vi "test_mean_map_filtered_M_stripped.vi"() -> ()   [LabVIEW 2009]
doc: "Copyright (C) 2009, Stepan A. Baranov\nweb: http://www.OCTLab.org/\nemail: stepan@baranov.su"
uses:
  OCTLib.dll
panel:
  out "min":dbl format="%0.2f"
  out "max":dbl format="%0.2f"
  out "version":string
  out "name":string
  out "error out":errorcluster
  out "offset":i32
  out "strip size":i32
  out "A-scan size":i32
  out "# of A-scans":i32
  in  "Small/Big":bool
  out "loop #":i32
  out "RSM_STAT time":u32
  out "LabView time":u32
  out "RSM_STAT Array":dbl[][](array[numeric])
  out "LabView Array":dbl[][](array[numeric])
  in  "stop":bool
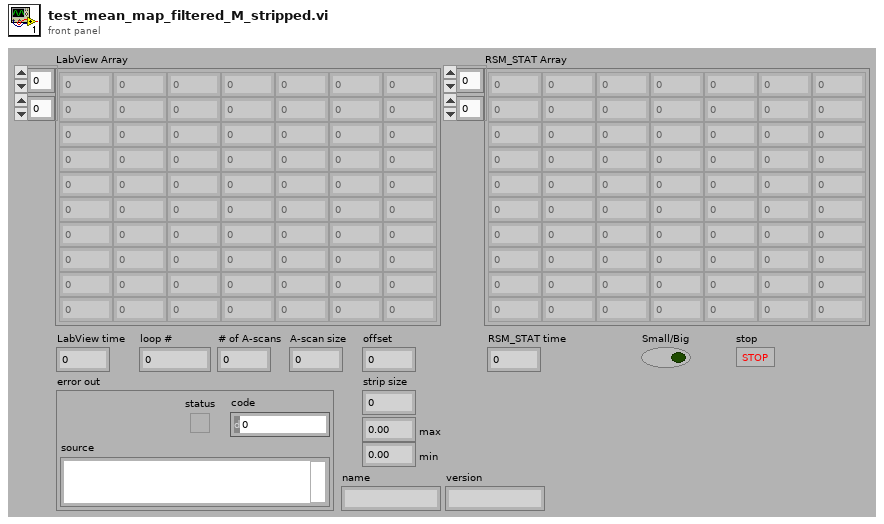
[diagram p1: front panel]
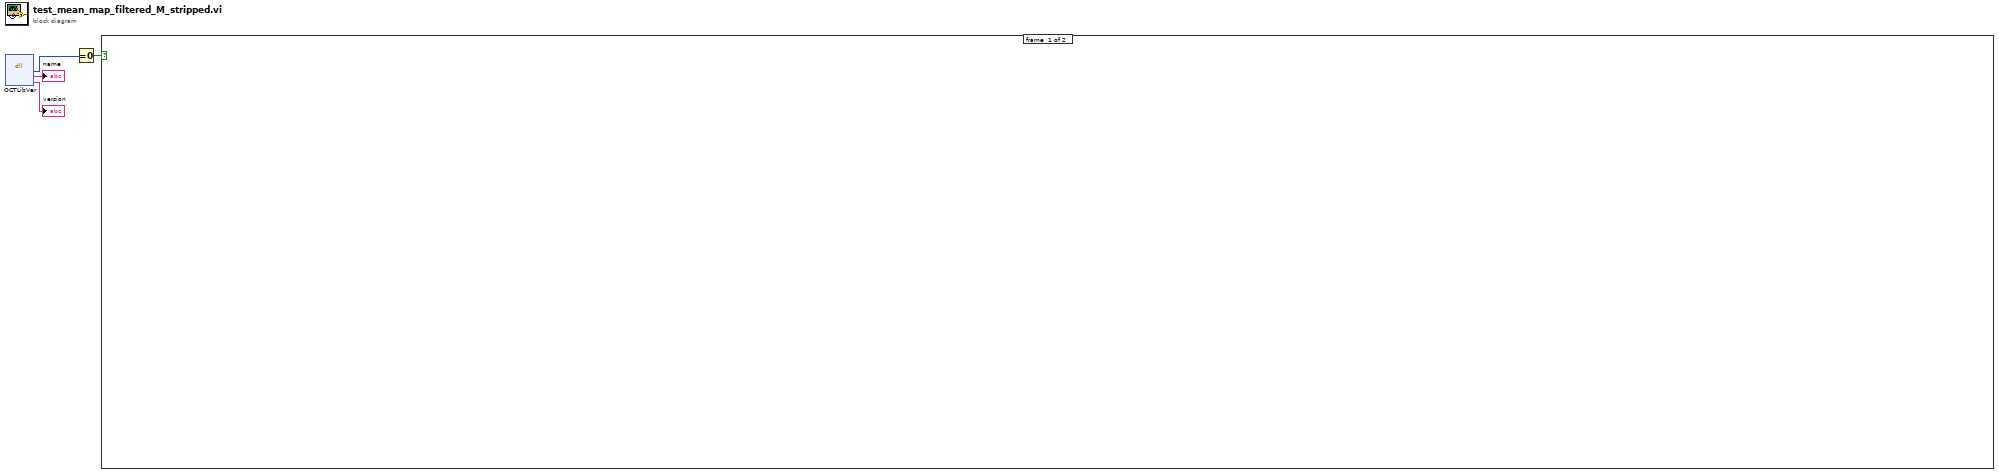
[diagram p0: block diagram]
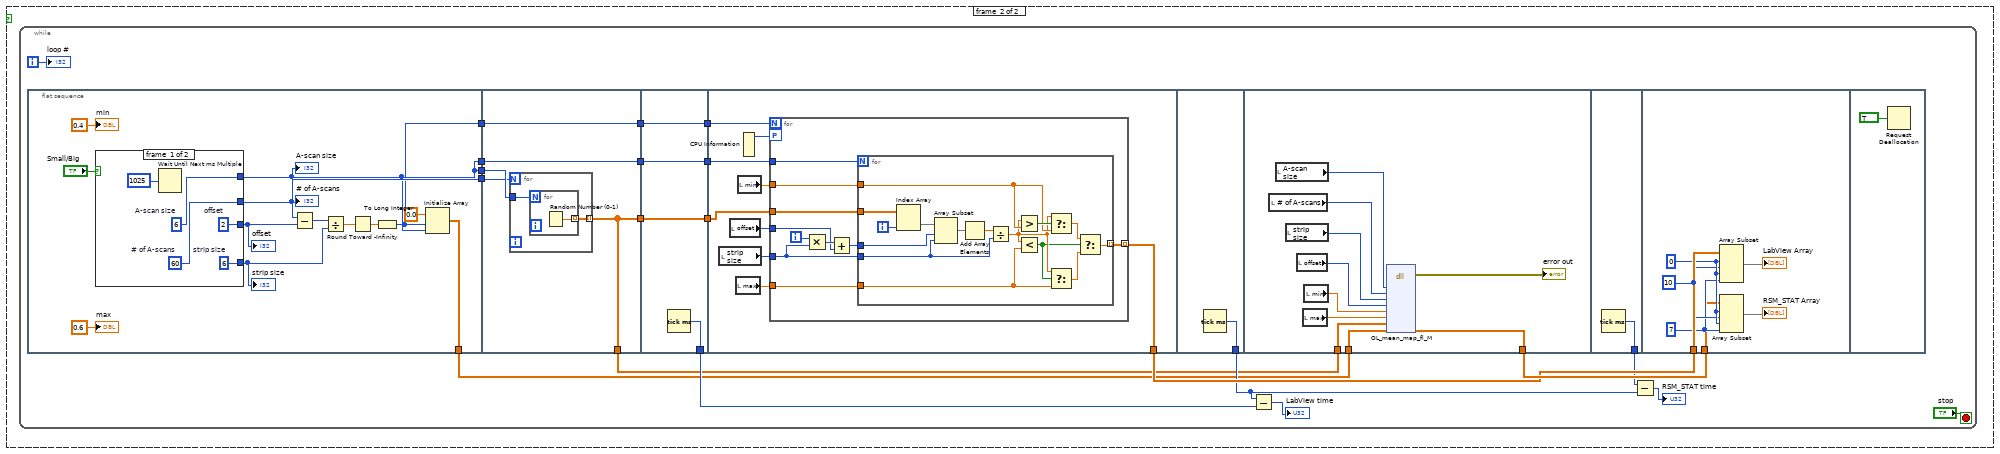
[diagram p2: hidden frame]
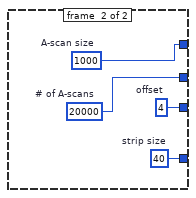
[diagram p3: hidden frame]
diagram:
  n1 = dll-call lib="OCTLib.dll" fn="OCTLibVer"() -> ("status"=w4:i8, "name"=→"name":string, "version"=→"version":string)  [unwired: 5 in, 2 out]
  n2 = Equal To 0?(x=w4) -> (x = 0?=w3:bool)
  n3 = case shown="True" w3 {
    frame #0 {
    }
    frame #1 {
      n4 = while {
        i -> [w17]
        stop <- "stop" stop-if-true
        n5 = flat-sequence {
          tunnel: [w32] -> w13
          tunnel: [w37] -> w12
          tunnel: [w35] -> w11
          tunnel: [w26] -> w6
          tunnel: [w32] -> w5
          tunnel: [w52] -> w16
          tunnel: [w52] -> w14
          tunnel: w13 -> [w51]
          tunnel: w12 -> [w50]
          tunnel: [w48] -> w10
          tunnel: [w49] -> w8
          tunnel: w6 -> [w49]
          tunnel: w5 -> [w48]
          tunnel: [w59] -> w22
          tunnel: [w58] -> w15
          tunnel: w14 -> [w58]
          tunnel: w10 -> [w57]
          tunnel: [w57] -> w9
          tunnel: w8 -> [w56]
          tunnel: [w56] -> w7
          tunnel: [w67] -> w23
          tunnel: w15 -> [w63]
          tunnel: w9 -> [w66]
          tunnel: w7 -> [w65]
          tunnel: [w94] -> w19
          tunnel: w16 -> [w101]
          tunnel: [w104] -> w24
          tunnel: w11 -> [w100]
          tunnel: [w105] -> w20
          tunnel: w24 -> [w106]
          tunnel: w23 -> [w112]
          frame #0 {
            n6 = case shown="False" "Small/Big" {
              tunnel: [w42 w46] -> w37
              tunnel: [w43 w47] -> w32
              tunnel: [w40 w45] -> w29
              tunnel: [w39 w44] -> w31
              frame #0 {
                w39 = 2  # offset
                w40 = 6  # strip size
                w43 = 6  # A-scan size
                w42 = 60  # # of A-scans
                n7 = Wait Until Next ms Multiple(millisecond multiple=u32 1025) -> ()  [unwired: 1 out]
              }
              frame #1 {
                w44 = 4  # offset
                w45 = 40  # strip size
                w47 = 1000  # A-scan size
                w46 = 20000  # # of A-scans
              }
            }
            "# of A-scans" <- w37
            "A-scan size" <- w32
            "strip size" <- w29
            "offset" <- w31
            n8 = Subtract(x=w37, y=w31) -> (x-y=w30:i32)
            n9 = Divide(x=w30, y=w29) -> (x/y=w28:dbl)
            n10 = Round Toward -Infinity(1:w28) -> (0:w27:dbl)
            n11 = To Long Integer(number=w27) -> (32bit integer=w26:i32)
            n12 = Initialize Array(0.0 ("element"), w26, w32) -> (w35:dbl[][])
            "max" <- 0.6 ("min")
            "min" <- 0.4 ("min")
          }
          frame #1 {
            n13 = for {
              N: w50 -> [_]
              tunnel: w51 -> [w54]
              tunnel: [w53] -> w52 mode=indexing
              n14 = for {
                N: w54 -> [_]
                tunnel: [w55] -> w53 mode=indexing
                n15 = Random Number (0-1)() -> (number: 0 to 1=w55:dbl)
              }
            }
          }
          frame #2 {
            n16 = Tick Count (ms)() -> (millisecond timer value=w59:u32)
          }
          frame #3 {
            n17 = local read "strip size"() -> (w60:i32)
            n18 = local read "offset"() -> (w64:i32)
            n19 = local read "max"() -> (w61:dbl)
            n20 = CPU Information() -> (4:w68:i32)  [unwired: 3 out]
            n21 = local read "min"() -> (w62:dbl)
            n22 = for {
              N: w65 -> [_]
              tunnel: [w78] -> w67 mode=indexing
              workers-P: w68 -> [_]
              tunnel: w66 -> [w77]
              tunnel: w60 -> [w72]
              tunnel: w64 -> [w70]
              tunnel: w63 -> [w76]
              tunnel: w62 -> [w75]
              tunnel: w61 -> [w74]
              i -> [w73]
              n23 = Multiply(x=w73, y=w72) -> (x*y=w71:i32)
              n24 = Add(x=w71, y=w70) -> (x+y=w69:i32)
              n25 = for {
                N: w77 -> [_]
                tunnel: w69 -> [w89]
                tunnel: [w93] -> w78 mode=indexing
                tunnel: w72 -> [w86]
                tunnel: w76 -> [w92]
                tunnel: w75 -> [w84]
                tunnel: w74 -> [w82]
                i -> [w91]
                n26 = Index Array(array=w92, index (col)=w91) -> (element=w90:dbl[])  [unwired: 1 in]
                n27 = Array Subset(array=w90, index=w89, length=w86) -> (w88:dbl[])
                n28 = Add Array Elements(numeric array=w88) -> (sum=w87:dbl)
                n29 = Divide(x=w87, y=w86) -> (x/y=w83:dbl)
                n30 = Greater?(x=w83, y=w84) -> (0:w85:bool)
                n31 = Less?(x=w83, y=w82) -> (x < y?=w81:bool)
                n32 = Select(t=w83, s=w85, f=w84) -> (s? t:f=w80:dbl)
                n33 = Select(t=w83, s=w81, f=w82) -> (s? t:f=w79:dbl)
                n34 = Select(t=w80, s=w81, f=w79) -> (s? t:f=w93:dbl)
              }
            }
          }
          frame #4 {
            n35 = Tick Count (ms)() -> (millisecond timer value=w94:u32)
          }
          frame #5 {
            n36 = local read "# of A-scans"() -> (w102:i32)
            n37 = local read "A-scan size"() -> (w103:i32)
            n38 = local read "strip size"() -> (w95:i32)
            n39 = local read "offset"() -> (w96:i32)
            n40 = local read "max"() -> (w97:dbl)
            n41 = local read "min"() -> (w98:dbl)
            n42 = dll-call lib="OCTLib.dll" fn="OL_mean_map_fl_M"("A-scan size"=w103, "# of A-scan"=w102, "strip size"=w95, "offset"=w96, "min"=w98, "max"=w97, "input"=w101, "data"=w100) -> (error out=→"error out":errorcluster, "data"=w104:dbl[][])  [unwired: 11 in, 1 out]
          }
          frame #6 {
            n43 = Tick Count (ms)() -> (millisecond timer value=w105:u32)
          }
          frame #7 {
            w109 = 10 ("length")
            w108 = 7 ("length")
            w110 = 0 ("index")
            n44 = Array Subset(array=w112, index (row)=w110, length (row)=w109, index (col)=w110, length (col)=w108) -> (→"LabView Array":dbl[][])
            n45 = Array Subset(array=w106, index (row)=w110, length (row)=w109, index (col)=w110, length (col)=w108) -> (→"RSM_STAT Array":dbl[][])
          }
          frame #8 {
            n46 = Request Deallocation(TRUE ("flag")) -> ()
          }
        }
        n47 = Subtract(x=w19, y=w22) -> (x-y=→"LabView time":u32)
        n48 = Subtract(x=w20, y=w19) -> (x-y=→"RSM_STAT time":u32)
        "loop #" <- w17
      }
    }
  }
